vi "质控模块润洗OK命令.vi"(8 "error in (no error)":errorcluster, 11 "质控润洗OK":bool) -> (0 "error out":errorcluster)   [LabVIEW 2016, in "质控单元V1.lvlib"]
uses:
  <vilib>/Plasmionique/MB Master/MB Master.lvlib
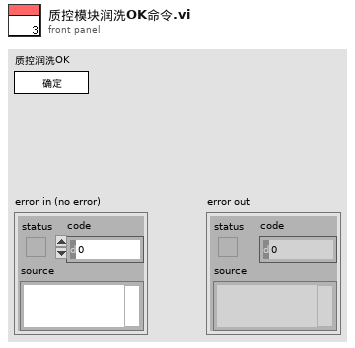
[diagram p1: front panel]
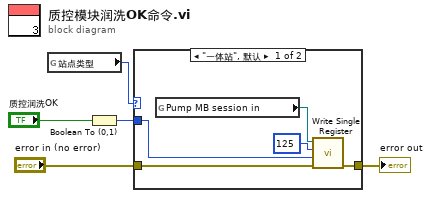
[diagram p0: block diagram]
diagram:
  n1 = global read "系统交互.vi" "站点类型"() -> (w4:enum16{"一体站", "固定站", "浮船", "一体站V1-V3", "养殖渭水"})
  n2 = Boolean To (0,1)(Boolean="质控润洗OK") -> (0, 1=w3:i16)
  n3 = case shown="\"一体站\", 默认" w4 {
    tunnel: w3 -> [w8 _]
    tunnel: "error in (no error)" -> [w7 w11]
    tunnel: [w6 w11] -> w1
    frame "一体站", Default {
      n4 = global read "系统交互.vi" "Pump MB session in"() -> (w9:refnum<class "MB_Master.lvclass">)
      n5 = call <vilib>:"Write Single Register.vi"("error in (no error)"=w7, "value"=w8, "address"=u16 125 ("starting address"), "MB session in"=w9) -> ("error out"=w6:errorcluster)  [unwired: 6 in, 1 out]
    }
    frame "养殖渭水" {
    }
  }
  "error out" <- w1
